vi "Close-GUI.vi"(8 "error in (no error)":errorcluster) -> (0 "error out":errorcluster)   [LabVIEW 2013, in "SLMServer.lvlib" / "SLMServer.lvclass"]
uses:
  SLMServer.lvclass
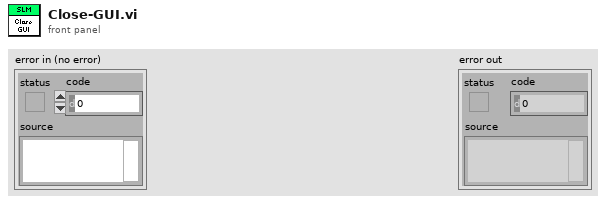
[diagram p1: front panel]
types:
  T1 = enum32{"invalid app kind", "Development System", "Run Time System", "Student Edition", "Embedded LabVIEW", "Evaluation", "Custom"}
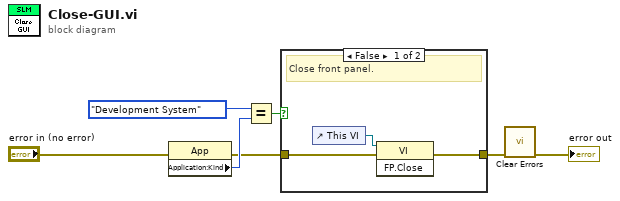
[diagram p0: block diagram]
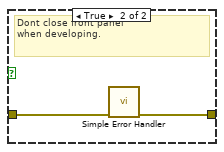
[diagram p2: hidden frame]
diagram:
  n1 = property on="Property Node" class="App"(error in="error in (no error)") -> (error out=w2:errorcluster, "Application:Kind"=w5:T1)  [unwired: 1 in, 1 out]
  n2 = Equal?(x=T1."Development System" ("y"), y=w5) -> (x = y?=w3:bool)
  n3 = case shown="False" w3 {
    tunnel: w2 -> [w9 w12]
    tunnel: [w8 w11] -> w1
    frame False {
      # "Close front panel."
      n4 = control-ref of="This VI"() -> (w10:refnum<vi>)
      n5 = invoke class="VI" method="FP.Close"(reference=w10, error in=w9) -> (error out=w8:errorcluster)  [unwired: 1 in, 2 out]
    }
    frame True {
      # "Dont close front panel\nwhen developing."
      n6 = call <vilib>:"Simple Error Handler.vi"("error in (no error)"=w12) -> ("error out"=w11:errorcluster)  [unwired: 4 in, 4 out]
    }
  }
  n7 = call <vilib>:"Clear Errors.vi"("error in (no error)"=w1) -> ("error out"=→"error out":errorcluster)  [unwired: 6 in]
